vi "Synchronize_Programs.vi"(3 "Mode":T6, 5 "Traverse line In":T3 {"Row Duration (mins)" format="%#.1f"; "Row No" min=0; "Trace Gas Concentration (%)" min=0.0 format="%#.2f"; "Emission Rate (l/min)" format="%#.2f"; "Tunnel Speed" format="%#.2f"; "Start X" format="%#.2f"; "Start Y" format="%#.2f"; "Start Z" format="%#.2f"; "End X" format="%#.2f"; "End Y" format="%#.2f"; "End Z" format="%#.2f"; "Averaging time (min)" min=0.0 format="%#.1f"}) -> (0 "Error Message":string, 1 "Status":T2, 2 "Traverse line Out":T3 {"Row Duration (mins)" format="%#.1f"; "Row No" min=0; "Trace Gas Concentration (%)" min=0.0 format="%#.2f"; "Emission Rate (l/min)" format="%#.2f"; "Tunnel Speed" format="%#.2f"; "Start X" format="%#.2f"; "Start Y" format="%#.2f"; "Start Z" format="%#.2f"; "End X" format="%#.2f"; "End Y" format="%#.2f"; "End Z" format="%#.2f"; "Averaging time (min)" min=0.0 format="%#.1f"})   [LabVIEW 2010]
uses:
  Gen Trav/Traverse_cluster.ctl
  Gen Trav/Spacing.ctl
  Controls/Multi_run_mode.ctl
  Controls/User_Specific_mode.ctl
  Gen Trav/Multi_Run_Status.ctl
  Gen Trav/Sync_Program_Case.ctl
  Controls/In_Range.ctl
  ADAM Client/Sub VIs/ADAM Controls/Update_scan_value.ctl
  ADAM Client/Sub VIs/ADAM Controls/Channel_State.ctl
  ADAM Client/Sub VIs/ADAM Controls/Client_Source_Status.ctl
  Globals/Preference_global.vi
  Globals/Meas_global.vi
panel:
  out "Is this the first Sync?":bool
  in  "Continue without sync":bool
  in  "stop":bool
  out "Has gas been switched off?":bool
  out "Has error email been sent?":bool
  out "Raise alarm after (mins)":i32
  out "Jump to fall back row if partner hung":bool
  out "Partners names":string[](array[string])
  out "Sync No":i32
  out "Sync Prog case":T1
  # "X           Y            Z"
  # "Start"
  # "End"
  # "X           Y            Z"
  # "Start"
  # "End"
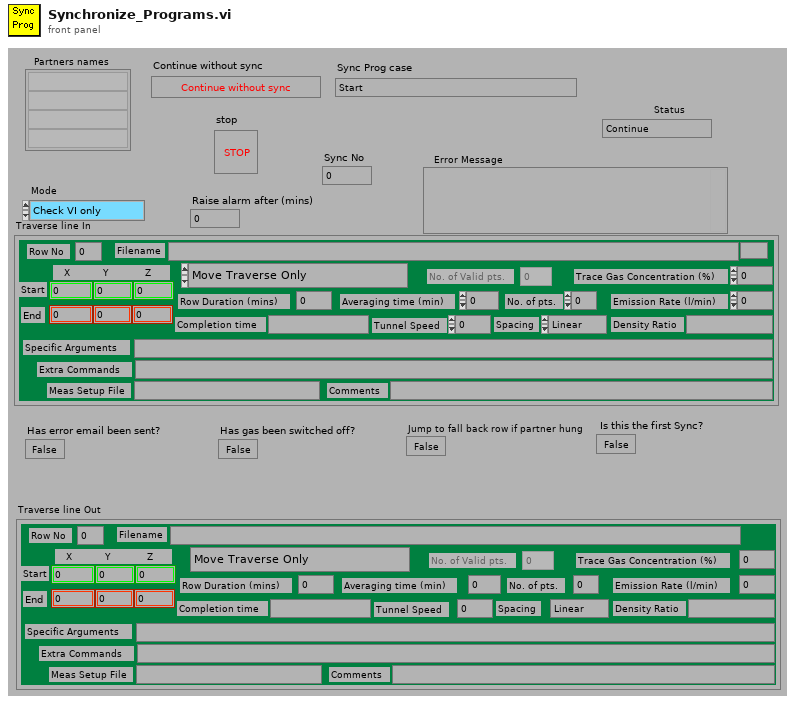
[diagram p1: front panel]
types:
  T1 = typedef "Sync_Program_Case.ctl" = enum16{"Start", "Is current Sync Number more than 2 minutes old?", "Publish Program State", "Find out about Partners", "Wait for partners to catch up", "End"}
  T2 = typedef "Multi_Run_Status.ctl" = enum16{"Continue", "Jump to Next Point", "Jump to Next Row", "Jump To Fall Back", "Terminate Run"}
  T3 = typedef "Traverse_cluster.ctl" = cluster{"Start X":dbl, "Start Y":dbl, "Start Z":dbl, "End X":dbl, "End Y":dbl, "End Z":dbl, "No. of pts.":i32, "Spacing":T4, "Filename":path, "Tunnel Speed":dbl, "Averaging time (min)":dbl, "Extra Commands":string, "Specific Arguments":string, "Emission Rate (l/min)":dbl, "Trace Gas Concentration (%)":dbl, "Density Ratio":string, "Comments":string, "Row No":i32, "Row Type Selector":T5, "Completion time":string, "Row Duration (mins)":dbl, "No. of Valid pts.":i32, "Meas Setup File":string}
  T4 = typedef "Spacing.ctl" = enum16{"Linear", "Log", "Gauss", "Specified", "N/A"}
  T5 = typedef "Multi_run_mode.ctl" = enum16{"Move Traverse Only", "Set Tunnel Speed Only", "Set Source Only", "Set Measurement Conditions", "Single Measurement", "Vertical Profile", "Lateral Profile", "Longitudinal Profile", "Explore Volume", "Multi-Axis Profile", "Auto Calibrate", "Meas Fast FID Bkgnd", "Check Beam Power", "Scanning Valve Measurement", "Run VI Named:", "Set ADAM Ch", "Wait (minutes)", "Send Message", "Synchronize With:", "Fall Back to this Row", "Turn Off Row Repeating", "Blank Row"}
  T6 = typedef "User_Specific_mode.ctl" = enum16{"Check VI only", "Run VI"}
  T7 = typedef "In_Range.ctl" = enum16{"%", "±", "% & ±"}
  T8 = typedef "Update_scan_value.ctl" = cluster{"Channel Name":string, "New Value":dbl}
  T9 = typedef "Channel_State.ctl" = enum16{"On", "Off", "Always On", "Always Off"}
  T10 = typedef "Client_Source_Status.ctl" = enum16{"Not Using", "Using", "Must Have"}
  T11 = typedef "Ch_description_ADAM.ctl" = cluster{"Ch Name":string, "Type":T12, "Function":T13, "Ch State":T9, "Calibration type":T14, "A":dbl, "B":dbl, "C":dbl, "D":dbl, "Comments":string, "Address":T15, "String":string, "Duty":u16}
  T12 = typedef "Module_type_ADAM.ctl" = enum16{"4011", "4012", "4013", "4014", "4016", "4017", "4018", "4021", "4050", "4052", "4053", "4060", "4080", "5000", "5017", "5018", "5024", "5051", "5056", "5060", "6060", "Tracker", "WEST", "GILL", "JEM", "VICI", "Vaisala", "DRUCK", "Run VI Named:", "IR2100", "PPT", "Comparator", "VIRTUAL", "Hold Value", "Read A", "Read Ch", "Coded", "Client Info", "Web Client", "X10", "Test"}
  T13 = typedef "Function_ADAM.ctl" = enum16{"Analogue Input", "Digital Input", "Event counter", "Event rate", "Analogue Output", "Digital Output", "Relay Output"}
  T14 = typedef "Calib_type_ADAM.ctl" = enum16{"Raw", "Bx + A", "Cx^2 + Bx + A", "Dx^3 + Cx^2 + Bx + A", "In Band", "Hi-Tec Q", "Hi-Tec M_dot", "Text"}
  T15 = typedef "Address.ctl" = cluster{"Main":i32, "Ch.":i32, "Sub":i32, "Port Name":string}
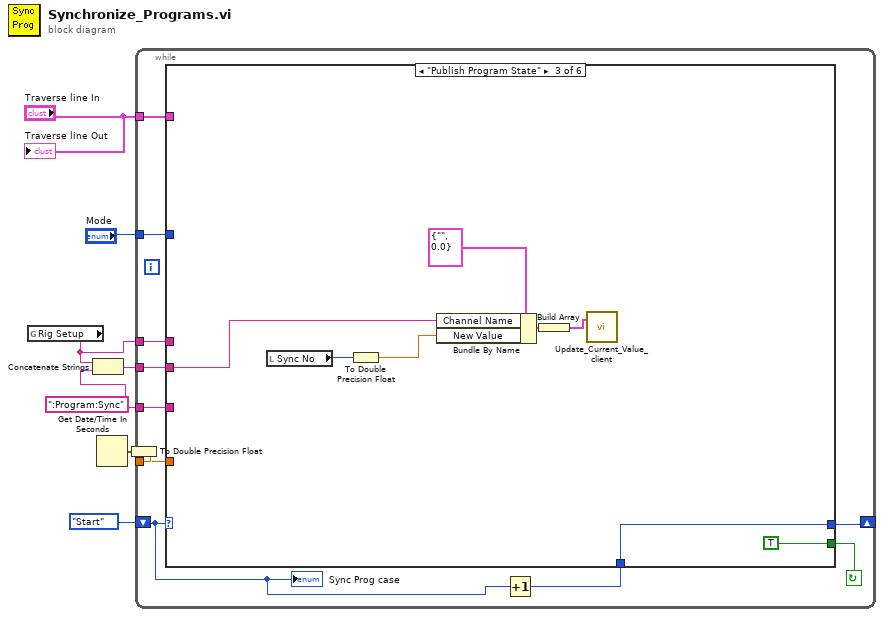
[diagram p0: block diagram]
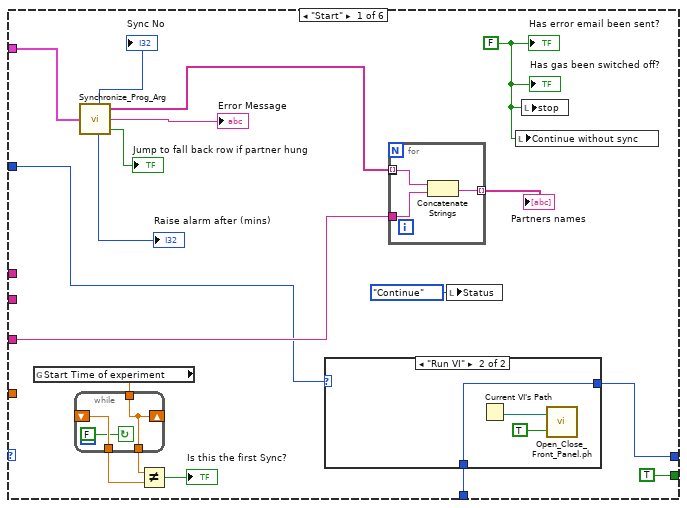
[diagram p2: hidden frame]
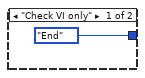
[diagram p3: hidden frame]
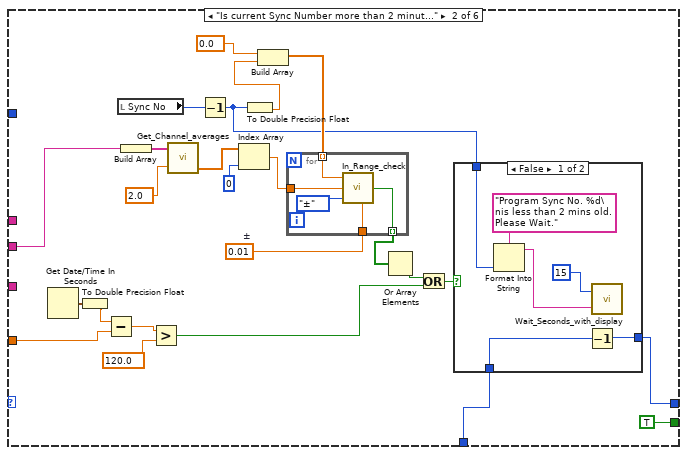
[diagram p4: hidden frame]
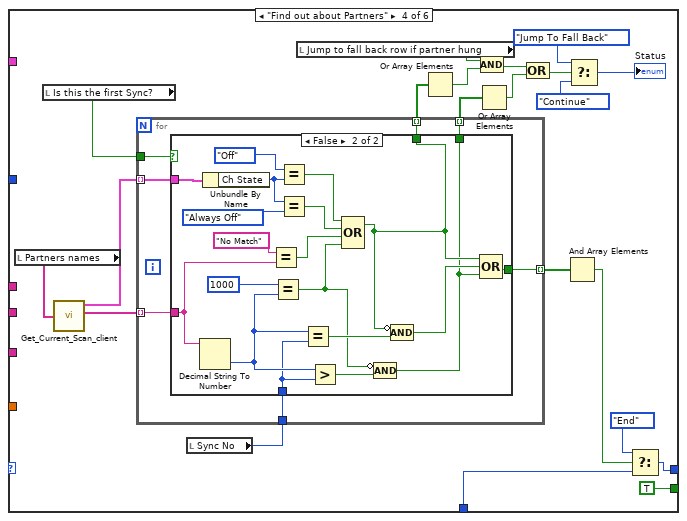
[diagram p6: hidden frame]
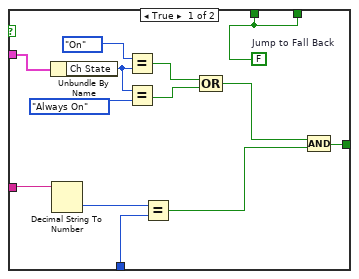
[diagram p7: hidden frame]
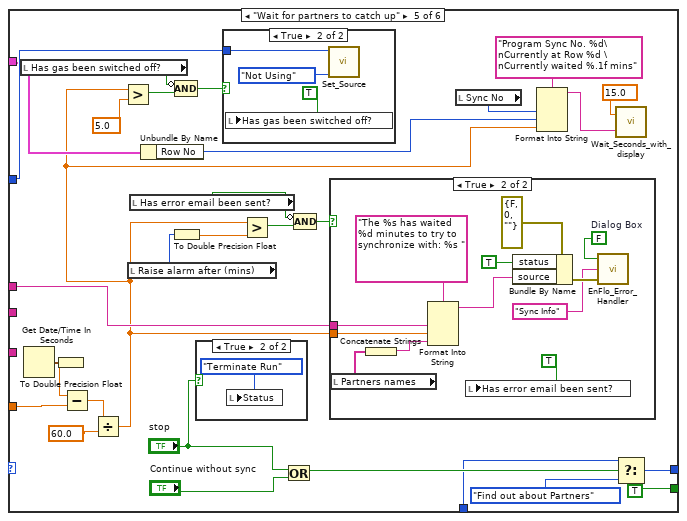
[diagram p8: hidden frame]
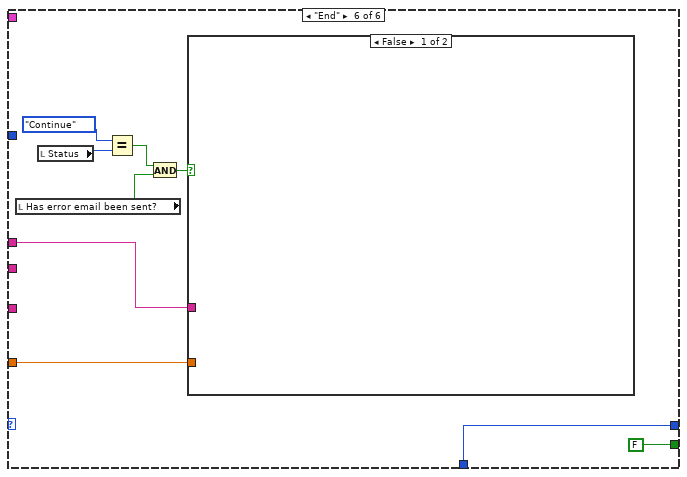
[diagram p12: hidden frame]
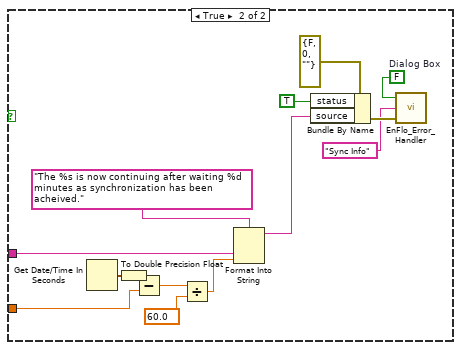
[diagram p13: hidden frame]
diagram:
  w4 = ":Program:Sync"
  n1 = global read "Preference_global.vi" "Rig Setup"() -> (w2:string)
  n2 = Concatenate Strings(w2, w4) -> (w3:string)
  n3 = Get Date/Time In Seconds() -> (seconds since 1Jan1904=w1:timestamp)
  n4 = To Double Precision Float(number=w1) -> (double precision float=w5:dbl)
  n5 = while {
    tunnel: w2 -> [w9]
    tunnel: w5 -> [w10]
    tunnel: w3 -> [w11]
    tunnel: w4 -> [w12]
    tunnel: "Mode" -> [w15]
    tunnel: "Traverse line In" -> [w16]
    shift-left: Sync_Program_Case."Start" ("Sync Prog case") -> [w17]
    shift-right: [w14] -> _
    stop <- w18 continue-if-true
    n6 = Increment(x=w17) -> (x+1=w13:T1)
    n7 = case shown="\"Publish Program State\"" w17 {
      tunnel: [TRUE TRUE TRUE TRUE TRUE FALSE] -> w18
      tunnel: w16 -> [w29 _ _ _ w155 _]
      tunnel: w15 -> [w19 _ _ _ w171 _]
      tunnel: [w32 w64 w84 w106 w160 w204] -> w14
      tunnel: w13 -> [w30 w63 w84 w107 w161 w204]
      tunnel: w12 -> [w26 _ _ _ _ _]
      tunnel: w11 -> [_ w69 w83 _ _ _]
      tunnel: w10 -> [_ w59 _ _ w178 w203]
      tunnel: w9 -> [_ _ _ _ w165 w200]
      frame "Start" {
        w24 = FALSE
        n8 = global read "Meas_global.vi" "Start Time of experiment"() -> (w22:dbl)
        n9 = while {
          tunnel: [w38] -> w20
          tunnel: [w39] -> w21
          tunnel: w22 -> [w39]
          shift-left: _ -> [w38]
          shift-right: [w39] -> _
          stop <- FALSE continue-if-true
        }
        n10 = call "Synchronize_Prog_Arg.vi"("Execution Row"=w29) -> ("Jump to fall back row"=→"Jump to fall back row if partner hung":bool, "Raise alarm after (mins)"=→"Raise alarm after (mins)":i32, "Error Comments"=→"Error Message":string, "Machine names"=w27:string[], "Sync No"=→"Sync No":i32)
        n11 = Not Equal?(x=w21, y=w20) -> (x != y?=→"Is this the first Sync?":bool)
        n12 = case shown="\"Run VI\"" w19 {
          tunnel: [Sync_Program_Case."End" ("Sync Prog case") w46] -> w32
          tunnel: w30 -> [_ w46]
          frame "Check VI only" {
          }
          frame "Run VI" {
            n13 = Current VI's Path() -> (path=w44:path)
            n14 = call "Open_Close_Front_Panel.ph.vi"("Front Panel Window:Open"=TRUE, "VI path"=w44) -> ()  [unwired: 1 in, 1 out]
          }
        }
        n15 = for {
          tunnel: [w40] -> _ mode=indexing
          tunnel: w26 -> [w42]
          tunnel: [w41] -> w28 mode=indexing
          tunnel: w27 -> [w40] mode=indexing
          n16 = Concatenate Strings(w40, w42) -> (w41:string)
        }
        "Partners names" <- w28
        n17 = local write "Status"(Multi_Run_Status."Continue" ("Status")) -> ()
        n18 = local write "Continue without sync"(w24) -> ()
        n19 = local write "stop"(w24) -> ()
        "Has error email been sent?" <- w24
        "Has gas been switched off?" <- w24
      }
      frame "Is current Sync Number more than 2 minutes old?" {
        w61 = 0.01  # ±
        n20 = Get Date/Time In Seconds() -> (seconds since 1Jan1904=w47:timestamp)
        n21 = To Double Precision Float(number=w47) -> (double precision float=w60:dbl)
        n22 = Subtract(x=w60, y=w59) -> (x-y=w58:dbl)
        n23 = local read "Sync No"() -> (w49:i32)
        n24 = Build Array(w69) -> (w68:string[])
        n25 = Greater?(x=w58, y=120.0) -> (0:w56:bool)
        n26 = call "Get_Channel_averages.vi"("Desired Ch Names"=w68, "Averaging time (mins)"=2.0) -> ("number"=w67:dbl[])  [unwired: 1 in, 2 out]
        n27 = Decrement(x=w49) -> (x-1=w48:i32)
        n28 = Index Array(array=w67, index=0 ("Index")) -> (element=w62:dbl)
        n29 = To Double Precision Float(number=w48) -> (double precision float=w53:dbl)
        n30 = Build Array(0.0 ("Averaging time (mins)"), w53) -> (w52:dbl[])
        n31 = for {
          tunnel: w62 -> [w75]
          tunnel: w61 -> [w73]
          tunnel: [w72] -> w51 mode=indexing
          tunnel: w52 -> [w71] mode=indexing
          n32 = call "In_Range_check.vi"("±"=w73, "Mode"=In_Range."±", "Value"=w75, "Setpoint"=w71) -> ("In Range"=w72:bool)  [unwired: 3 in]
        }
        n33 = Or Array Elements(Boolean array=w51) -> (logical OR=w50:bool)
        n34 = Or(x=w50, y=w56) -> (x .or. y?=w55:bool)
        n35 = case shown="False" w55 {
          tunnel: [w79 w82] -> w64
          tunnel: w63 -> [w80 w82]
          tunnel: w48 -> [w77 _]
          frame False {
            n36 = Format Into String(format string="Program Sync No. %d\nis less than 2 mins old. Please Wait." ("Format String"), w77) -> (resulting string=w76:string)  [unwired: 2 in, 1 out]
            n37 = Decrement(x=w80) -> (x-1=w79:T1)
            n38 = call "Wait_Seconds_with_display.vi"("Message"=w76, "Seconds to wait"=u32 15) -> ()  [unwired: 1 in, 1 out]
          }
          frame True {
          }
        }
      }
      frame "Publish Program State" {
        n39 = local read "Sync No"() -> (w86:i32)
        n40 = To Double Precision Float(number=w86) -> (double precision float=w85:dbl)
        n41 = Bundle By Name(cluster=T8 {"Channel Name"="", "New Value"=0.0} ("Update Scan Value Cluster"), "Channel Name"=w83, "New Value"=w85) -> (w89:T8)
        n42 = Build Array(w89) -> (w87:T8[])
        n43 = call "Update_Current_Value_client.vi"("Update array in"=w87) -> ()  [unwired: 1 in]
      }
      frame "Find out about Partners" {
        n44 = local read "Partners names"() -> (w101:string[])
        n45 = local read "Is this the first Sync?"() -> (w91:bool)
        n46 = call "Get_Current_Scan_client.vi"("ADAM Ch Names"=w101) -> ("Ch Description Array"=w99:T11[], "String values"=w100:string[])  [unwired: 1 in, 1 out]
        n47 = local read "Sync No"() -> (w111:i32)
        n48 = for {
          tunnel: w111 -> [w113]
          tunnel: w100 -> [w117] mode=indexing
          tunnel: [w118] -> w110 mode=indexing
          tunnel: [w115] -> w104 mode=indexing
          tunnel: w99 -> [w116] mode=indexing
          tunnel: [w114] -> w95 mode=indexing
          tunnel: w91 -> [w112]
          n49 = case shown="False" w112 {
            tunnel: [w121 w150] -> w118
            tunnel: w117 -> [w124 w142]
            tunnel: w116 -> [w128 w141]
            tunnel: [w120 w138] -> w115
            tunnel: w113 -> [w119 w135]
            tunnel: [w120 w132] -> w114
            frame True {
              w120 = FALSE  # Jump to Fall Back
              n50 = Unbundle By Name(w128) -> ("Ch State"=w130:T9)
              n51 = Decimal String To Number(string=w124) -> (number=w125:i32)  [unwired: 2 in, 1 out]
              n52 = Equal?(x=Channel_State."On" ("Ch State"), y=w130) -> (x = y?=w127:bool)
              n53 = Equal?(x=w130, y=Channel_State."Always On" ("Ch State")) -> (x = y?=w126:bool)
              n54 = Equal?(x=w125, y=w119) -> (x = y?=w123:bool)
              n55 = Compound Arithmetic op=OR(w127, w126) -> (w122:bool)
              n56 = Compound Arithmetic op=AND(w122, w123) -> (w121:bool)
            }
            frame False {
              n57 = Decimal String To Number(string=w142) -> (number=w136:i32)  [unwired: 2 in, 1 out]
              n58 = Unbundle By Name(w141) -> ("Ch State"=w147:T9)
              n59 = Equal?(x="No Match", y=w142) -> (x = y?=w143:bool)
              n60 = Equal?(x=1000, y=w136) -> (x = y?=w133:bool)
              n61 = Equal?(x=Channel_State."Off" ("Ch State"), y=w147) -> (x = y?=w145:bool)
              n62 = Equal?(x=w147, y=Channel_State."Always Off" ("Ch State")) -> (x = y?=w144:bool)
              n63 = Equal?(x=w136, y=w135) -> (x = y?=w139:bool)
              n64 = Greater?(x=w136, y=w135) -> (0:w134:bool)
              n65 = Compound Arithmetic op=OR(w145, w144, w143, w133) -> (w138:bool)
              n66 = Compound Arithmetic op=AND(invert w133, w134) -> (w132:bool)
              n67 = Compound Arithmetic op=AND(invert w138, w139) -> (w140:bool)
              n68 = Compound Arithmetic op=OR(w138, w140, w132) -> (w150:bool)
            }
          }
        }
        n69 = local read "Jump to fall back row if partner hung"() -> (w102:bool)
        n70 = Or Array Elements(Boolean array=w104) -> (logical OR=w103:bool)
        n71 = Or Array Elements(Boolean array=w95) -> (logical OR=w93:bool)
        n72 = Compound Arithmetic op=AND(w102, w103) -> (w94:bool)
        n73 = Compound Arithmetic op=OR(w94, w93) -> (w92:bool)
        n74 = And Array Elements(Boolean array=w110) -> (logical AND=w109:bool)
        n75 = Select(t=Multi_Run_Status."Jump To Fall Back" ("Status"), s=w92, f=Multi_Run_Status."Continue" ("Status")) -> (s? t:f=→"Status":T2)
        n76 = Select(t=Sync_Program_Case."End" ("Sync Prog case"), s=w109, f=w107) -> (s? t:f=w106:T1)
      }
      frame "Wait for partners to catch up" {
        n77 = local read "Has gas been switched off?"() -> (w173:bool)
        n78 = Get Date/Time In Seconds() -> (seconds since 1Jan1904=w151:timestamp)
        n79 = To Double Precision Float(number=w151) -> (double precision float=w179:dbl)
        n80 = Subtract(x=w179, y=w178) -> (x-y=w177:dbl)
        n81 = Divide(x=w177, y=60.0) -> (x/y=w154:dbl)
        n82 = Greater?(x=w154, y=5.0) -> (0:w174:bool)
        n83 = local read "Raise alarm after (mins)"() -> (w167:i32)
        n84 = local read "Has error email been sent?"() -> (w169:bool)
        n85 = Unbundle By Name(w155) -> ("Row No"=w156:i32)
        n86 = To Double Precision Float(number=w167) -> (double precision float=w166:dbl)
        n87 = Compound Arithmetic op=AND(invert w173, w174) -> (w172:bool)
        n88 = case shown="True" "stop" {
          frame False {
          }
          frame True {
            n89 = local write "Status"(Multi_Run_Status."Terminate Run" ("Status")) -> ()
          }
        }
        n90 = case shown="True" w172 {
          tunnel: w171 -> [_ w195]
          frame False {
          }
          frame True {
            n91 = local write "Has gas been switched off?"(TRUE ("Has gas been switched off?")) -> ()
            n92 = call "Set_Source.vi"("Source Status"=Client_Source_Status."Not Using", "Simulate/Run"=w195) -> ()  [unwired: 2 in, 6 out]
          }
        }
        n93 = Greater?(x=w154, y=w166) -> (0:w168:bool)
        n94 = Or(x="stop", y="Continue without sync") -> (x .or. y?=w163:bool)
        n95 = Compound Arithmetic op=AND(invert w169, w168) -> (w170:bool)
        n96 = case shown="True" w170 {
          tunnel: w165 -> [_ w188]
          tunnel: w154 -> [_ w185]
          frame False {
          }
          frame True {
            w191 = FALSE  # Dialog Box
            n97 = local read "Partners names"() -> (w187:string[])
            n98 = Concatenate Strings(w187) -> (w184:string)
            n99 = Format Into String(format string="The %s has waited %d minutes to try to synchronize with: %s " ("Format String"), w188, w185, w184) -> (resulting string=w183:string)  [unwired: 2 in, 1 out]
            n100 = local write "Has error email been sent?"(TRUE ("Has gas been switched off?")) -> ()
            n101 = Bundle By Name(cluster=errorcluster {"status"=FALSE, "code"=0, "source"=""} ("error in (no error)"), "status"=TRUE ("Bundle Element"), "source"=w183) -> (w192:errorcluster)
            n102 = call "EnFlo_Error_Handler.vi"("error in (no error)"=w192, "Error Type"="Sync Info", "Dialog Box (T)"=w191) -> ()  [unwired: 3 out]
          }
        }
        n103 = local read "Sync No"() -> (w158:i32)
        n104 = Format Into String(format string="Program Sync No. %d\nCurrently at Row %d \nCurrently waited %.1f mins" ("Format String"), w158, w156, w154) -> (resulting string=w157:string)  [unwired: 2 in, 1 out]
        n105 = call "Wait_Seconds_with_display.vi"("Message"=w157, "Seconds to wait"=15.0) -> ()  [unwired: 1 in, 1 out]
        n106 = Select(t=w161, s=w163, f=Sync_Program_Case."Find out about Partners" ("Sync Prog case")) -> (s? t:f=w160:T1)
      }
      frame "End" {
        n107 = local read "Has error email been sent?"() -> (w202:bool)
        n108 = local read "Status"() -> (w199:T2)
        n109 = Equal?(x=Multi_Run_Status."Continue" ("Status"), y=w199) -> (x = y?=w197:bool)
        n110 = And(x=w197, y=w202) -> (x .and. y?=w201:bool)
        n111 = case shown="False" w201 {
          tunnel: w200 -> [_ w219]
          tunnel: w203 -> [_ w217]
          frame False {
          }
          frame True {
            w211 = FALSE  # Dialog Box
            n112 = Get Date/Time In Seconds() -> (seconds since 1Jan1904=w206:timestamp)
            n113 = To Double Precision Float(number=w206) -> (double precision float=w218:dbl)
            n114 = Subtract(x=w218, y=w217) -> (x-y=w216:dbl)
            n115 = Divide(x=w216, y=60.0) -> (x/y=w214:dbl)
            n116 = Format Into String(format string="The %s is now continuing after waiting %d minutes as synchronization has been acheived." ("Format String"), w219, w214) -> (resulting string=w207:string)  [unwired: 2 in, 1 out]
            n117 = Bundle By Name(cluster=errorcluster {"status"=FALSE, "code"=0, "source"=""} ("error in (no error)"), "status"=TRUE ("Bundle Element"), "source"=w207) -> (w212:errorcluster)
            n118 = call "EnFlo_Error_Handler.vi"("error in (no error)"=w212, "Error Type"="Sync Info", "Dialog Box (T)"=w211) -> ()  [unwired: 3 out]
          }
        }
      }
    }
    "Sync Prog case" <- w17
  }
  "Traverse line Out" <- "Traverse line In"
